vi "rotate_1d_array_roi.vi"(7 "rotate?":T1, 11 "array in":dbl[](array[numeric])) -> (3 "array out":dbl[](array[numeric]))   [LabVIEW 2010]
uses:
  rotate_controller.ctl
  SignalWriterMH110203USBStepperMotor.lvclass
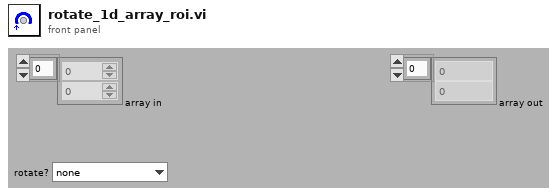
[diagram p1: front panel]
types:
  T1 = typedef "SignalWriterMH110203USBStepperMotor.lvclass/rotate_controller.ctl" = enum16{"none", "90", "180", "270", "mirror horizontal"}
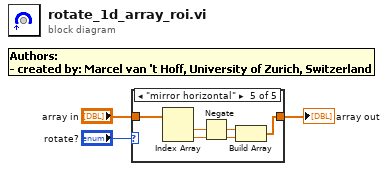
[diagram p0: block diagram]
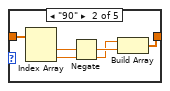
[diagram p3: hidden frame]
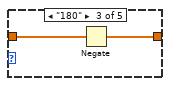
[diagram p4: hidden frame]
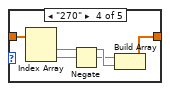
[diagram p5: hidden frame]
diagram:
  n1 = case shown="\"mirror horizontal\"" "rotate?" {
    tunnel: "array in" -> [w4 w9 w11 w16 w21]
    tunnel: [w4 w5 w10 w15 w17] -> w1
    frame "none", Default {
    }
    frame "90" {
      n2 = Index Array(array=w9) -> (element #1=w8:dbl, element #2=w6:dbl)  [unwired: 2 in]
      n3 = Negate(x=w8) -> (-x=w7:dbl)
      n4 = Build Array(w6, w7) -> (w5:dbl[])
    }
    frame "180" {
      n5 = Negate(x=w11) -> (-x=w10:dbl[])
    }
    frame "270" {
      n6 = Index Array(array=w16) -> (element #1=w14:dbl, element #2=w13:dbl)  [unwired: 2 in]
      n7 = Negate(x=w13) -> (-x=w12:dbl)
      n8 = Build Array(w12, w14) -> (w15:dbl[])
    }
    frame "mirror horizontal" {
      n9 = Index Array(array=w21) -> (element #1=w20:dbl, element #2=w18:dbl)  [unwired: 2 in]
      n10 = Negate(x=w20) -> (-x=w19:dbl)
      n11 = Build Array(w19, w18) -> (w17:dbl[])
    }
  }
  "array out" <- w1
